vi "Set Parameter.vi"(8 "error in (no error)":errorcluster, 10 "Parameter":refnum<class "AbstractData.lvclass">, 11 "SolarSystems M266 Old in":refnum<class "SolarSystems M266 Old.lvclass">) -> (0 "error out":errorcluster, 3 "SolarSystems M266 Old out":refnum<class "SolarSystems M266 Old.lvclass">)   [LabVIEW 2014, in "SolarSystems M266 Old.lvclass"]
uses:
  SolarSystems M266 Old.lvclass
  Framework/Model/Data/AbstractData/AbstractData.lvclass
  SolarSystems M266 Old.lvclass/SolarSystems M266 Old.ctl
  Framework/Model/Data/DataSingleElement/DataSingleElement.lvclass
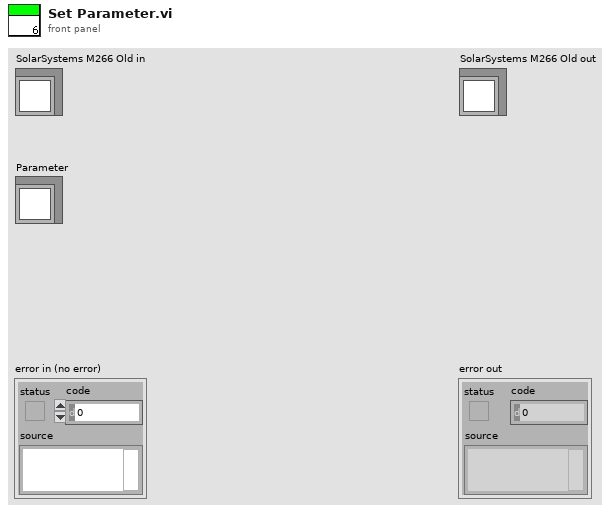
[diagram p1: front panel]
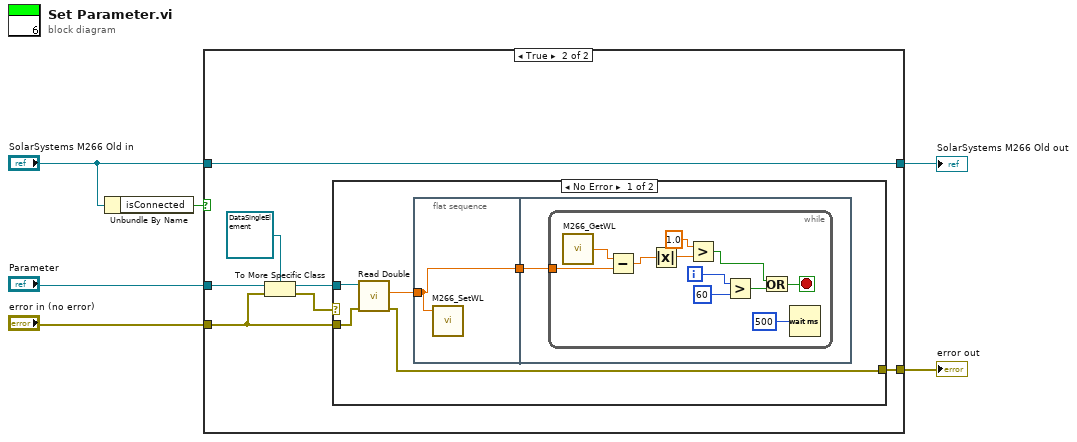
[diagram p0: block diagram]
diagram:
  n1 = Unbundle By Name("SolarSystems M266 Old in") -> ("isConnected"=w6:bool)
  n2 = case shown="True" w6 {
    tunnel: [w7 w10] -> w4
    tunnel: "error in (no error)" -> [w7 w12]
    tunnel: [w8 w15] -> w5
    tunnel: "SolarSystems M266 Old in" -> [w8 w15]
    tunnel: "Parameter" -> [_ w14]
    frame False {
    }
    frame True {
      n3 = To More Specific Class(target class=refnum<class "DataSingleElement.lvclass"> refnum ("DataSingleElement.lvclass"), reference=w14, error in=w12) -> (specific class reference=w9:refnum<class "DataSingleElement.lvclass">, error out=w11:errorcluster)
      n4 = case shown="No Error" w11 {
        tunnel: w12 -> [w19 w34]
        tunnel: [w18 w34] -> w10
        tunnel: w9 -> [w20 _]
        frame No Error {
          n5 = call "Read Double.vi"("error in (no error)"=w19, "DataSingleElement in"=w20) -> ("error out"=w18:errorcluster, "value"=w17:dbl)  [unwired: 7 in, 1 out]
          n6 = flat-sequence {
            tunnel: w17 -> [w21]
            tunnel: [w21] -> w16
            tunnel: w16 -> [w22]
            frame #0 {
              n7 = call "M266_SetWL.vi"("WL"=w21) -> ()  [unwired: 2 in, 1 out]
            }
            frame #1 {
              n8 = while {
                tunnel: w22 -> [w28]
                i -> [w32]
                stop <- w29 stop-if-true
                n9 = call "M266_GetWL.vi"() -> ("Current WL"=w23:dbl)
                n10 = Subtract(x=w23, y=w28) -> (x-y=w27:dbl)
                n11 = Absolute Value(x=w27) -> (abs(x)=w26:dbl)
                n12 = Greater?(x=1.0, y=w26) -> (0:w24:bool)
                n13 = Greater?(x=w32, y=60) -> (0:w30:bool)
                n14 = Or(x=w24, y=w30) -> (x .or. y?=w29:bool)
                n15 = Wait (ms)(milliseconds to wait=u32 500) -> ()  [unwired: 1 out]
              }
            }
          }
        }
        frame Error {
        }
      }
    }
  }
  "error out" <- w4
  "SolarSystems M266 Old out" <- w5
